vi "EnchantedRoomParams.vi"(8 "error in (no error)":errorcluster, 11 "EnchantedRoom":refnum<class "EnchantedRoom.lvclass">) -> (0 "error out":errorcluster, 2 "EnchantedRoomParams":T1, 3 "EnchantedRoom":refnum<class "EnchantedRoom.lvclass">)   [LabVIEW 2020, in "EnchantedRoom.lvclass"]
uses:
  EnchantedRoom.lvclass
  TypeDef/EnchantedRoomParams.ctl
  Spell/Spell.lvclass
  EnchantedRoom.lvclass/EnchantedRoom.ctl
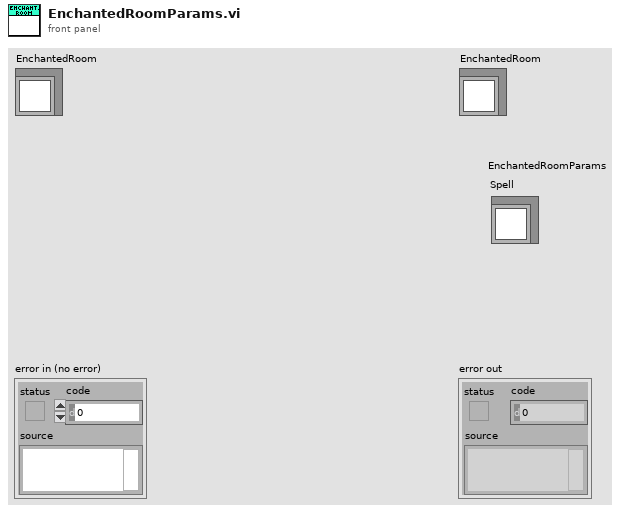
[diagram p1: front panel]
types:
  T1 = typedef "EnchantedRoom.lvclass/EnchantedRoomParams.ctl" = cluster{"Spell":refnum<class "Spell.lvclass">}
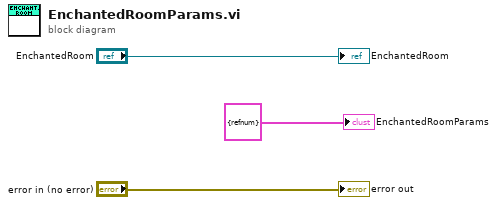
[diagram p0: block diagram]
diagram:
  "error out" <- "error in (no error)"
  "EnchantedRoom" <- "EnchantedRoom"
  "EnchantedRoomParams" <- T1 {"Spell"=refnum} ("<ClassName>Params")
